vi "find tag mapped to channel.vi"(7 "owner":string, 8 "error in":errorcluster, 10 "action channel":refnum<class "TBM channel.lvclass">, 11 "engine configuration in":refnum<class "base TBM sequencer configuration.lvclass">) -> (0 "error out":errorcluster, 2 "seq channel":refnum<class "TBM channel.lvclass">, 3 "engine configuration out":refnum<class "base TBM sequencer configuration.lvclass">)   [LabVIEW 2014, in "base TBM sequencer configuration.lvclass"]
uses:
  base TBM sequencer configuration.lvclass
  <vilib>/NI/Tag Bus Module Framework/channel/TBM channel.lvclass
  <vilib>/NI/Configuration Framework/NISE_CEF_TreeControl.lvlib
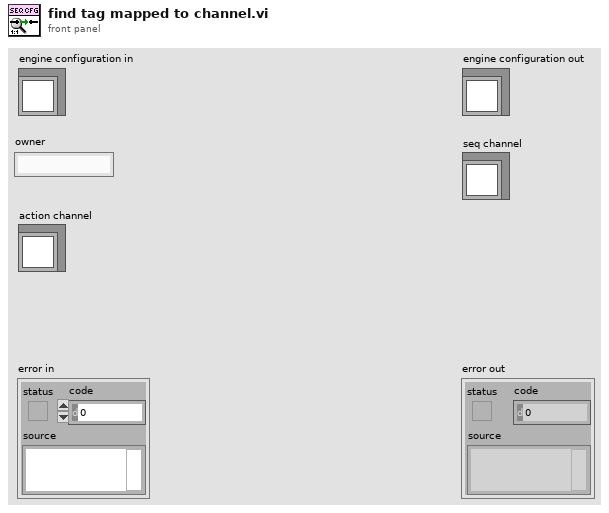
[diagram p1: front panel]
types:
  T1 = typedef "tag bus.lvlib/data table.lvlib/mapping specification.ctl" = cluster{"data type":T2, "mappings":T3[]}
  T2 = typedef "tag bus.lvlib/tag descriptor.lvclass/Data Type.ctl" = enum16{"Double", "Single", "I64", "I32", "I16", "I8", "U64", "U32", "U16", "U8", "Boolean", "String", "Array of Double", "Array of Single", "Array of I64", "Array of I32", "Array of I16", "Array of I8", "Array of U64", "Array of U32", "Array of U16", "Array of U8", "Array of Boolean", "Array of String"}
  T3 = typedef "tag bus.lvlib/data table.lvlib/mapping.ctl" = cluster{"sink name":string, "source name":string}
  T4 = typedef "TBM channel.lvclass/channel classification.ctl" = enum16{"input data", "output data", "processing parameter", "processing result"}
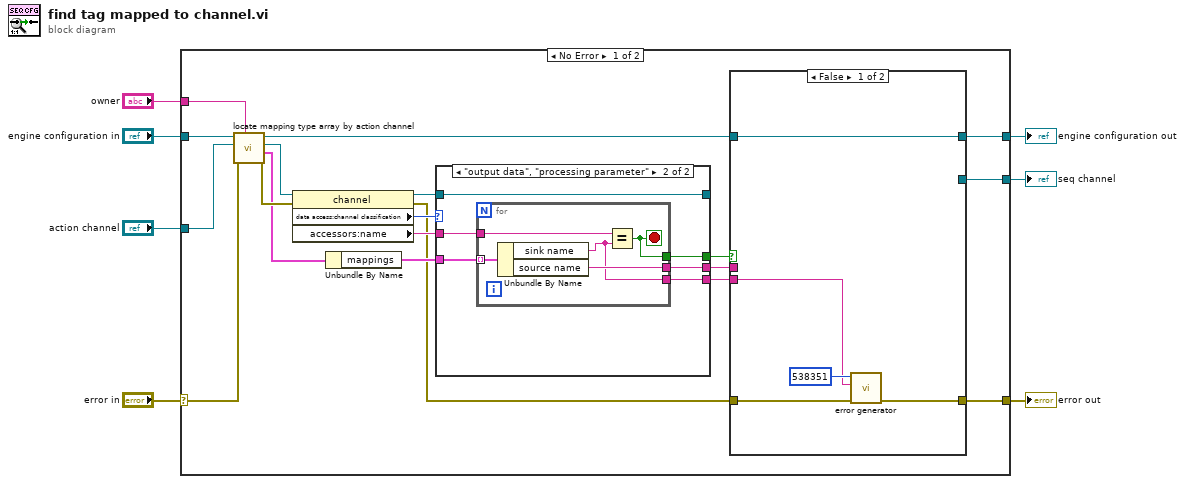
[diagram p0: block diagram]
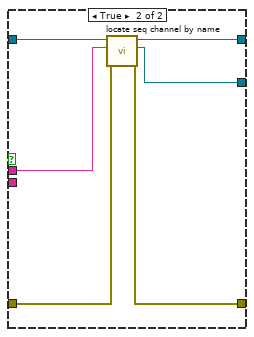
[diagram p2: hidden frame]
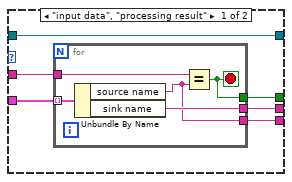
[diagram p3: hidden frame]
diagram:
  n1 = case shown="No Error" "error in" {
    selector: "error in" -> [w23 w61]
    tunnel: [w11 w61] -> w6
    tunnel: [w14 w60] -> w4
    tunnel: "engine configuration in" -> [w25 w60]
    tunnel: "owner" -> [w26 _]
    tunnel: "action channel" -> [w24 _]
    tunnel: [w9 _] -> w1
    frame No Error {
      n2 = call "locate mapping type array by action channel.vi"("owner ID"=w26, "error in"=w23, "action channel"=w24, "engine configuration in"=w25) -> ("error out"=w21:errorcluster, "Mapping"=w18:T1, "action channel out"=w22:refnum<class "TBM channel.lvclass">, "engine configuration out"=w15:refnum<class "base TBM sequencer configuration.lvclass">)  [unwired: 4 in]
      n3 = property class="channel"(reference=w22, error in=w21) -> (reference out=w20:refnum<class "TBM channel.lvclass">, error out=w10:errorcluster, "data access:channel classification"=w19:T4, "accessors:name"=w16:string)
      n4 = Unbundle By Name(w18) -> ("mappings"=w17:T3[])
      n5 = case shown="\"output data\", \"processing parameter\"" w19 {
        tunnel: w20 -> [w43 w54]
        tunnel: [w43 w54] -> _
        tunnel: w17 -> [w42 w52]
        tunnel: w16 -> [w41 w53]
        tunnel: [w40 w51] -> w12
        tunnel: [w39 w50] -> w13
        tunnel: [w38 w49] -> w8
        frame "input data", "processing result" {
          n6 = for {
            tunnel: w42 -> [w48] mode=indexing
            tunnel: w41 -> [w47]
            tunnel: [w46] -> w40
            tunnel: [w45] -> w39
            tunnel: [w44] -> w38
            stop <- w46 stop-if-true
            n7 = Unbundle By Name(w48) -> ("source name"=w44:string, "sink name"=w45:string)
            n8 = Equal?(x=w47, y=w44) -> (x = y?=w46:bool)
          }
        }
        frame "output data", "processing parameter" {
          n9 = for {
            tunnel: w52 -> [w59] mode=indexing
            tunnel: w53 -> [w58]
            tunnel: [w57] -> w51
            tunnel: [w56] -> w50
            tunnel: [w55] -> w49
            stop <- w57 stop-if-true
            n10 = Unbundle By Name(w59) -> ("sink name"=w55:string, "source name"=w56:string)
            n11 = Equal?(x=w58, y=w55) -> (x = y?=w57:bool)
          }
        }
      }
      n12 = case shown="False" w12 {
        tunnel: w15 -> [w31 w37]
        tunnel: [w31 w36] -> w14
        tunnel: w13 -> [_ w35]
        tunnel: [w27 w33] -> w11
        tunnel: w10 -> [w28 w34]
        tunnel: [_ w32] -> w9
        tunnel: w8 -> [w29 _]
        frame False {
          n13 = call <vilib>:"error generator.vi"("error in"=w28, "append error message"=w29, "error code (0)"=538351) -> ("error out"=w27:errorcluster)  [unwired: 6 in]
        }
        frame True {
          n14 = call "locate seq channel by name.vi"("error in"=w34, "channel name"=w35, "engine configuration in"=w37) -> ("error out"=w33:errorcluster, "channel descriptor"=w32:refnum<class "TBM channel.lvclass">, "engine configuration out"=w36:refnum<class "base TBM sequencer configuration.lvclass">)  [unwired: 6 in]
        }
      }
    }
    frame Error {
    }
  }
  "error out" <- w6
  "engine configuration out" <- w4
  "seq channel" <- w1
